vi "DATA TYPES.vi"() -> ()   [LabVIEW 2019]
panel:
  out "Boolean 2":bool
  in  "Boolean":bool
  out "CHARACTER 2":string
  in  "CHARACTER":string
  out "INTEGER 2":u8
  in  "INTEGER":u8
  out "Numeric 2":dbl
  in  "FLOAT":dbl
  # "DIFFERENT DATA TYPES"
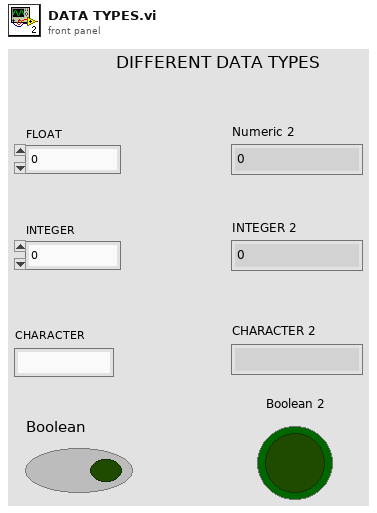
[diagram p1: front panel]
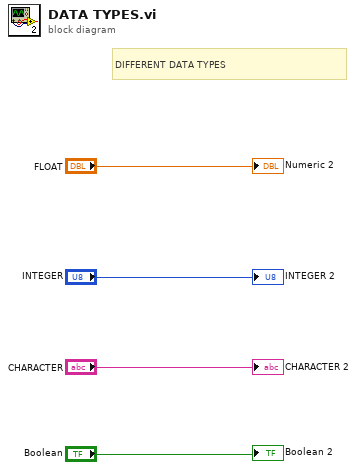
[diagram p0: block diagram]
diagram:
  # "DIFFERENT DATA TYPES"
  "Numeric 2" <- "FLOAT"
  "INTEGER 2" <- "INTEGER"
  "CHARACTER 2" <- "CHARACTER"
  "Boolean 2" <- "Boolean"
